vi "Create.vi"(6 "Overwrite?":bool, 8 "error in":errorcluster, 9 "SheetName":string="Sheet1", 10 "Path":path) -> (0 "error out":errorcluster, 3 "SpreadsheetDoc":refnum<k24>)   [LabVIEW 2019, in "Open Xml.lvlib"]
uses:
  Open Xml.lvlib
  D:/git/Open-Xml-LabVIEW/Source/DocumentFormat.OpenXml.dll
  DocumentFormat.OpenXml.dll
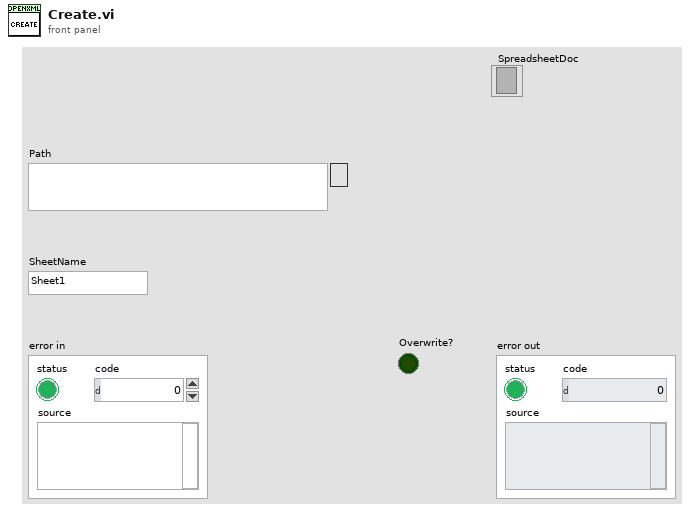
[diagram p1: front panel]
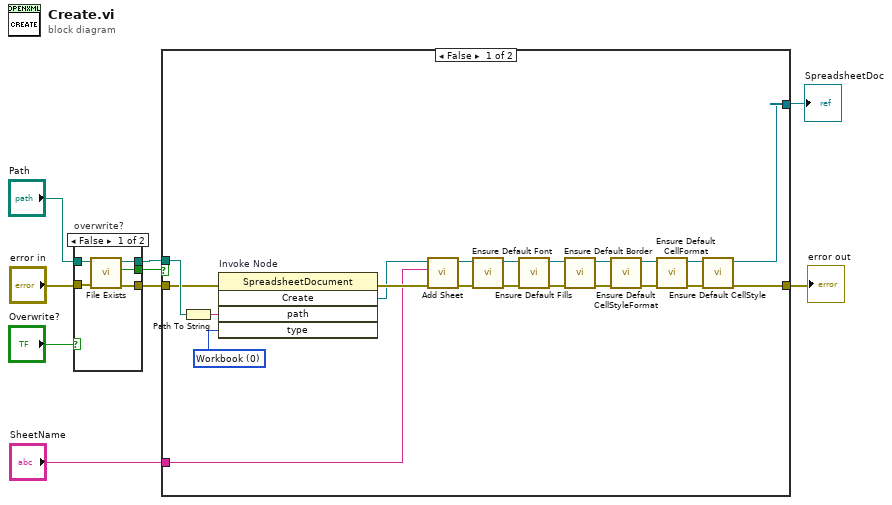
[diagram p0: block diagram]
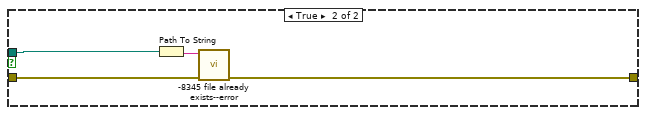
[diagram p2: hidden frame]
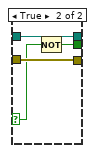
[diagram p3: hidden frame]
diagram:
  n1 = case "overwrite?" shown="False" "Overwrite?" {
    selector: "Overwrite?" -> [_ w16]
    tunnel: [w12 w15] -> w6
    tunnel: "error in" -> [w14 w18]
    tunnel: "Path" -> [w13 w17]
    tunnel: [w11 w17] -> w4
    tunnel: [w10 w18] -> w3
    frame False {
      n2 = call "File Exists.vi"("error in"=w14, "File Path"=w13) -> ("error out"=w10:errorcluster, "Exists"=w12:bool, "File Path (dup)"=w11:path)  [unwired: 7 in]
    }
    frame True {
      n3 = Not(x=w16) -> (.not. x?=w15:bool)
    }
  }
  n4 = case shown="False" w6 {
    tunnel: w4 -> [w39 w40]
    tunnel: w3 -> [w36 w43]
    tunnel: "SheetName" -> [w33 _]
    tunnel: [w30 _] -> w8
    tunnel: [w29 w42] -> w1
    frame False {
      w38 = 0 items=["Workbook", "Template", "MacroEnabledWorkbook", "MacroEnabledTemplate", "AddIn"] ("Type")
      n5 = Path To String(path=w39) -> (string=w37:string)
      n6 = invoke on="Invoke Node" class="SpreadsheetDocument" method="Create"(error in=w36, "path"=w37, "type"=w38) -> (error out=w35:errorcluster, "Create"=w34:refnum<k24>)  [unwired: 2 in, 3 out]
      n7 = call "Add Sheet.vi"("error in"=w35, "SheetName"=w33, "SpreadsheetDoc in"=w34) -> ("error out"=w31:errorcluster, "SpreadsheetDoc out"=w32:refnum<k24>)  [unwired: 7 in]
      n8 = call "Ensure Default Font.vi"("error in"=w31, "SpreadsheetDoc in"=w32) -> ("error out"=w28:errorcluster, "SpreadsheetDoc out"=w27:refnum<k24>)  [unwired: 8 in]
      n9 = call "Ensure Default Fills.vi"("error in"=w28, "SpreadsheetDoc in"=w27) -> ("error out"=w26:errorcluster, "SpreadsheetDoc out"=w25:refnum<k24>)  [unwired: 8 in]
      n10 = call "Ensure Default Border.vi"("error in"=w26, "SpreadsheetDoc in"=w25) -> ("error out"=w24:errorcluster, "SpreadsheetDoc out"=w23:refnum<k24>)  [unwired: 8 in]
      n11 = call "Ensure Default CellStyleFormat.vi"("error in"=w24, "SpreadsheetDoc in"=w23) -> ("error out"=w22:errorcluster, "SpreadsheetDoc out"=w21:refnum<k24>)  [unwired: 8 in]
      n12 = call "Ensure Default CellFormat.vi"("error in"=w22, "SpreadsheetDoc in"=w21) -> ("error out"=w20:errorcluster, "SpreadsheetDoc out"=w19:refnum<k24>)  [unwired: 8 in]
      n13 = call "Ensure Default CellStyle.vi"("error in"=w20, "SpreadsheetDoc in"=w19) -> ("error out"=w29:errorcluster, "SpreadsheetDoc out"=w30:refnum<k24>)  [unwired: 8 in]
    }
    frame True {
      n14 = Path To String(path=w40) -> (string=w41:string)
      n15 = call "-8345 file already exists--error.vi"("error in"=w43, "Argument"=w41) -> ("error out"=w42:errorcluster)  [unwired: 9 in]
    }
  }
  "SpreadsheetDoc" <- w8
  "error out" <- w1
